vi "Joystick Drive Control.vi"(10 "Arcade Drive?":bool, 11 "Cluster In":T11) -> ()   [LabVIEW 2018]
uses:
  <vilib>/Rock Robotics/WPI/MotorControl/WPI_MotorControlDeviceRef.ctl
  <vilib>/Rock Robotics/WPI/MotorControl/WPI_MotorControlType.ctl
  <vilib>/Rock Robotics/SystemInterfaces/DIO/FPGA_DIOPWMChannel.ctl
  <vilib>/Rock Robotics/WPI/PWM/WPI_PWMDeadband.ctl
  <vilib>/Rock Robotics/SystemInterfaces/DIO/FPGA_DIOChannel.ctl
  <vilib>/Rock Robotics/WPI/Joystick/WPI_JoystickDevRef.ctl
  <vilib>/Rock Robotics/WPI/Joystick/WPI_JoystickDeviceEnum.ctl
  <vilib>/Rock Robotics/WPI/DriverStation/WPI_DriverStationRobotMode2.ctl
  <vilib>/Rock Robotics/WPI/RobotDrive/WPI_RobotDriveDevRef.ctl
  Vision States.ctl
  <vilib>/Rock Robotics/WPI/ThirdParty/Phoenix-LabVIEW/Motor Controller/Controls/CTRE_Phoenix_MotorControl_ControlMode.ctl
  Robot Global Data.vi
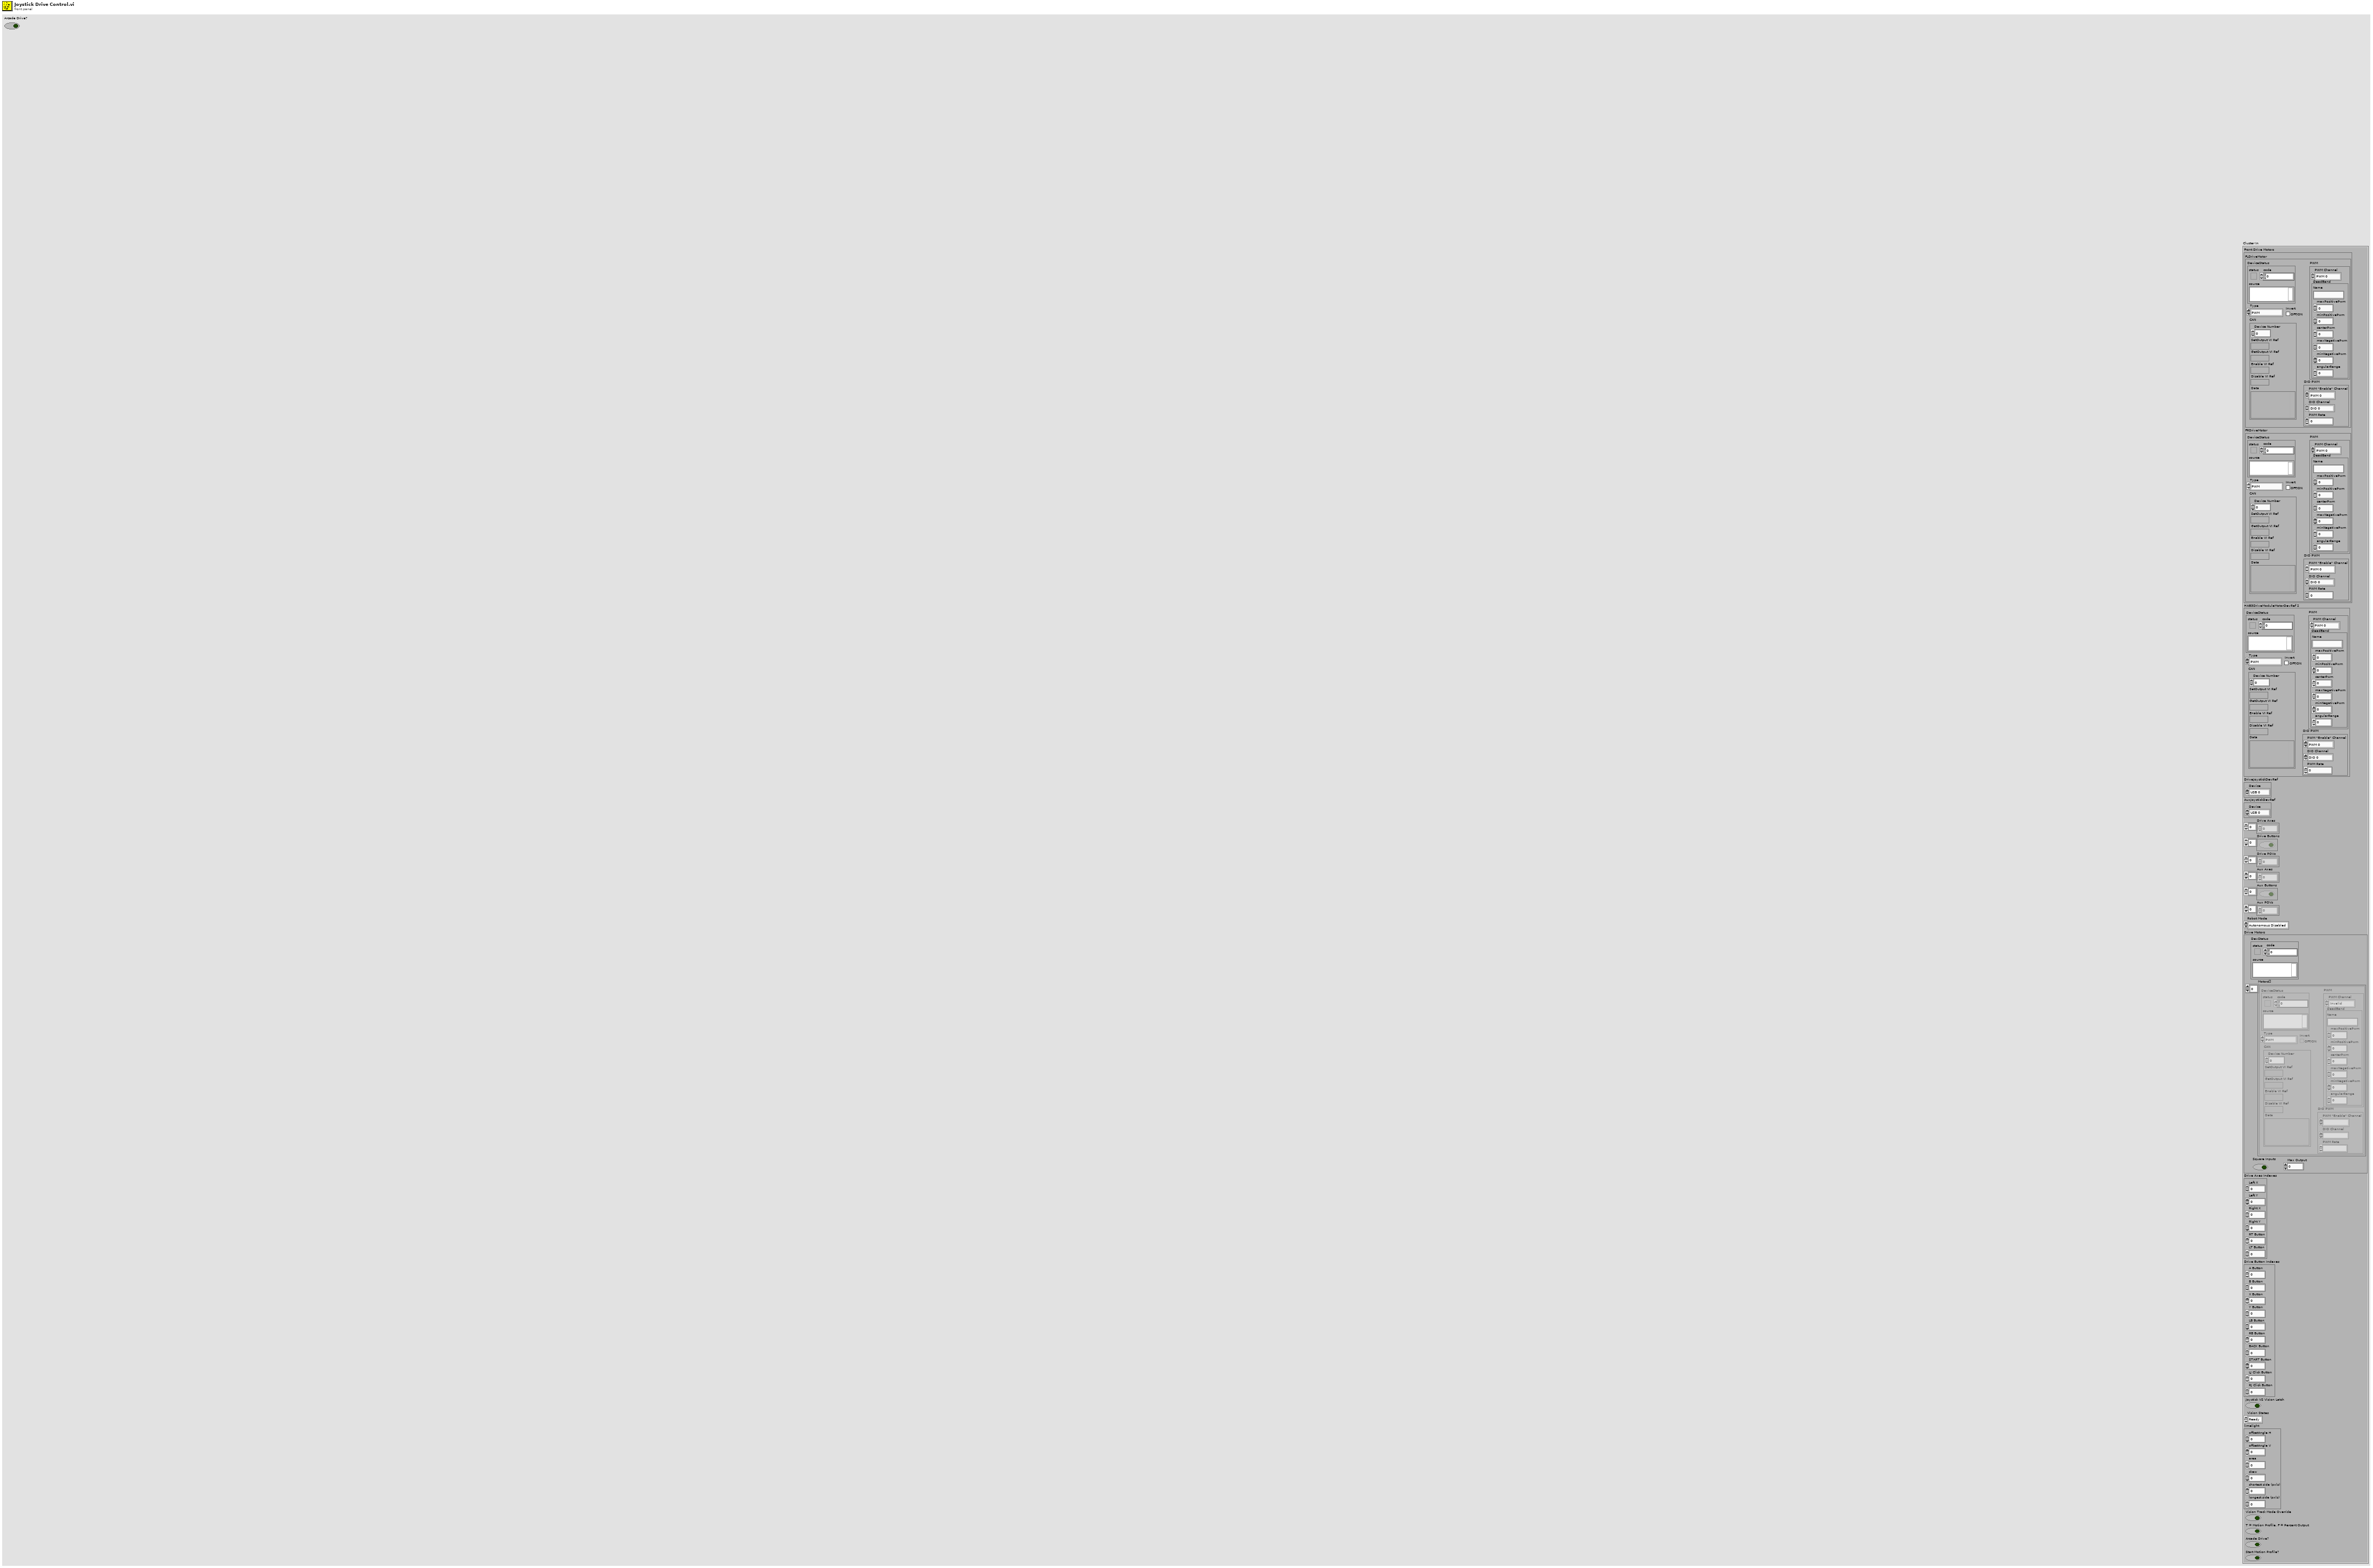
[diagram p1: front panel]
types:
  T1 = typedef "WPI_MotorControlDeviceRef.ctl" = cluster{"DeviceStatus":errorcluster, "Type":T2, "PWM":cluster{"PWM Channel":T3, "DeadBand":T4}, "CAN":cluster{"Device Number":u8, "SetOutput VI Ref":variant, "GetOutput VI Ref":variant, "Enable VI Ref":variant, "Disable VI Ref":variant, "Data":variant}, "Invert":bool, "DIO PWM":cluster{"PWM \"Enable\" Channel":T3, "DIOChannel":T5, "PWM Rate":dbl}}
  T2 = typedef "WPI_MotorControlType.ctl" = enum16{"PWM", "CAN", "DIO PWM"}
  T3 = typedef "FPGA_DIOPWMChannel.ctl" = enum8{"PWM 0", "PWM 1", "PWM 2", "PWM 3", "PWM 4", "PWM 5", "PWM 6", "PWM 7", "PWM 8", "PWM 9", "PWM MXP 0", "PWM MXP 1", "PWM MXP 2", "PWM MXP 3", "PWM MXP 4", "PWM MXP 5", "PWM MXP 6", "PWM MXP 7", "PWM MXP 8", "PWM MXP 9", "Invalid"}
  T4 = typedef "WPI_PWMDeadband.ctl" = cluster{"Name":string, "maxPositivePwm":i32, "minPositivePwm":i32, "centerPwm":i32, "maxNegativePwm":i32, "minNegativePwm":i32, "angularRange":u16}
  T5 = typedef "FPGA_DIOChannel.ctl" = enum8{"DIO 0", "DIO 1", "DIO 2", "DIO 3", "DIO 4", "DIO 5", "DIO 6", "DIO 7", "DIO 8", "DIO 9", "DIO MXP 0", "DIO MXP 1", "DIO MXP 2", "DIO MXP 3", "DIO MXP 4", "DIO MXP 5", "DIO MXP 6", "DIO MXP 7", "DIO MXP 8", "DIO MXP 9", "DIO MXP 10", "DIO MXP 11", "DIO MXP 12", "DIO MXP 13", "DIO MXP 14", "DIO MXP 15", "SPI Port CS1", "SPI Port CS2", "SPI Port CS3", "SPI Port MISO", "SPI Port MOSI", "Invalid"}
  T6 = typedef "WPI_JoystickDevRef.ctl" = cluster{"Device":T7}
  T7 = typedef "WPI_JoystickDeviceEnum.ctl" = enum16{"USB 0", "USB 1", "USB 2", "USB 3", "USB 4", "USB 5"}
  T8 = typedef "WPI_DriverStationRobotMode2.ctl" = enum16{"Autonomous Disabled", "Autonomous Enabled", "Teleop Disabled", "Teleop Enabled", "Disconnected", "Finish", "Test Disabled", "Test Enabled", "Emergency Stopped"}
  T9 = typedef "WPI_RobotDriveDevRef.ctl" = cluster{"DevStatus":errorcluster, "Motors[]":T1[], "Square Inputs":bool, "Max Output":dbl}
  T10 = typedef "Vision States.ctl" = enum16{"Ready", "Forward Until Target at Edge", "Vision Track"}
  T11 = cluster{"Front Drive Motors":cluster{"FLDriveMotor":T1, "FRDriveMotor":T1}, "HAB3DriveModuleMotorDevRef 2":T1, "DriveJoystickDevRef":T6, "AuxJoystickDevRef":T6, "Drive Axes":dbl[], "Drive Buttons":bool[], "Drive POVs":i16[], "Aux Axes":dbl[], "Aux Buttons":bool[], "Aux POVs":i16[], "Robot Mode":T8, "Drive Motors":T9, "Drive Axes Indexes":cluster{"Left X":i32, "Left Y":i32, "Right X":i32, "Right Y":i32, "RT Button":i32, "LT Button":i32}, "Drive Button Indexes":cluster{"A Button":i32, "B Button":i32, "X Button":i32, "Y Button":i32, "LB Button":i32, "RB Button":i32, "BACK Button":i32, "START Button":i32, "LJ Click Button":i32, "RJ Click Button":i32}, "Joystick VS Vision Latch":bool, "Vision States":T10, "limelight":cluster{"offsetAngle H":dbl, "offsetAngle V":dbl, "area":dbl, "skew":dbl, "shortest side (pxls)":dbl, "longest side (pxls)":dbl}, "Vision Track Mode Override":bool, "T = Motion Profile, F = Percent Output":bool, "Arcade Drive?":bool, "Start Motion Profile?":bool}
  T12 = typedef "CTRE_Phoenix_MotorControl_ControlMode.ctl" = u16
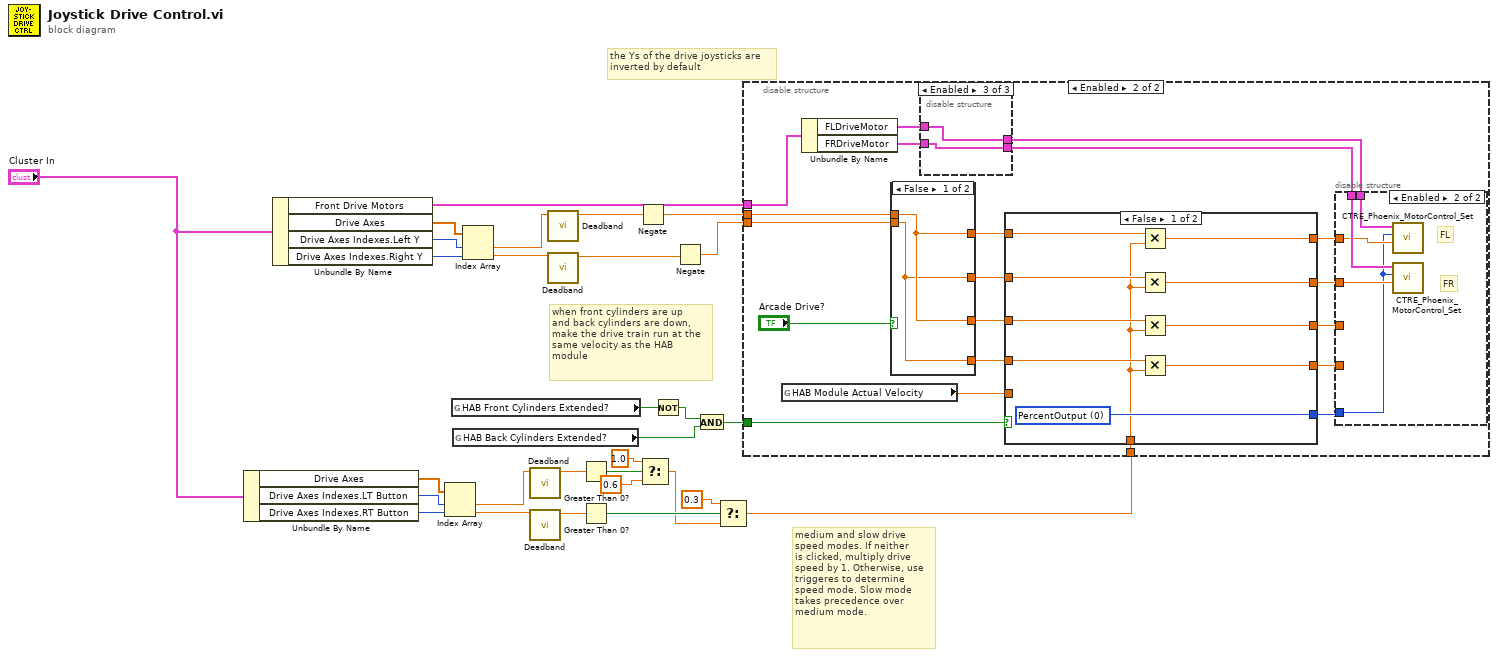
[diagram p0: block diagram]
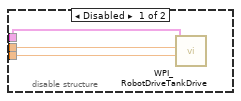
[diagram p2: hidden frame]
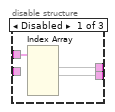
[diagram p3: hidden frame]
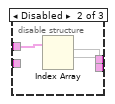
[diagram p4: hidden frame]
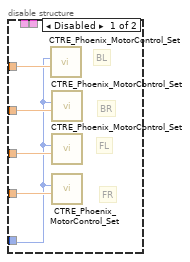
[diagram p5: hidden frame]
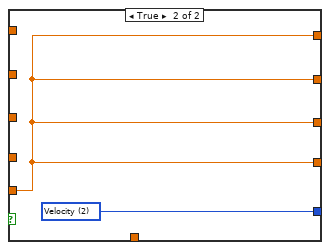
[diagram p7: hidden frame]
diagram:
  # "medium and slow drive\nspeed modes. If neither\nis clicked, multiply drive\nspeed by 1. Otherwise, use\ntriggeres to determine \nspeed mode. Slow mode\ntakes precedence over \nmedium mode."
  # "when front cylinders are up\nand back cylinders are down,\nmake the drive train run at the\nsame velocity as the HAB \nmodule"
  # "the Ys of the drive joysticks are \ninverted by default"
  n1 = Unbundle By Name("Cluster In") -> ("Drive Axes"=w13:dbl[], "Drive Axes Indexes.LT Button"=w14:i32, "Drive Axes Indexes.RT Button"=w15:i32)
  n2 = Unbundle By Name("Cluster In") -> ("Front Drive Motors"=w20:cluster{"FLDriveMotor":T1, "FRDriveMotor":T1}, "Drive Axes"=w21:dbl[], "Drive Axes Indexes.Left Y"=w22:i32, "Drive Axes Indexes.Right Y"=w23:i32)
  n3 = Index Array(array=w13, index #1=w14, index #2=w15) -> (element #1=w12:dbl, element #2=w16:dbl)
  n4 = global read "Robot Global Data.vi" "HAB Front Cylinders Extended?"() -> (w19:bool)
  n5 = global read "Robot Global Data.vi" "HAB Back Cylinders Extended?"() -> (w2:bool)
  n6 = Index Array(array=w21, index #1=w22, index #2=w23) -> (element #1=w26:dbl, element #2=w27:dbl)
  n7 = call "Deadband.vi"("Input"=w12) -> ("Output"=w11:dbl)  [unwired: 10 in]
  n8 = call "Deadband.vi"("Input"=w16) -> ("Output"=w10:dbl)  [unwired: 10 in]
  n9 = call "Deadband.vi"("Input"=w26) -> ("Output"=w29:dbl)  [unwired: 10 in]
  n10 = call "Deadband.vi"("Input"=w27) -> ("Output"=w28:dbl)  [unwired: 10 in]
  n11 = Greater Than 0?(x=w11) -> (x > 0?=w8:bool)
  n12 = Greater Than 0?(x=w10) -> (x > 0?=w9:bool)
  n13 = Negate(x=w29) -> (-x=w25:dbl)
  n14 = Select(t=1.0, s=w8, f=0.6) -> (s? t:f=w5:dbl)
  n15 = Not(x=w19) -> (.not. x?=w18:bool)
  n16 = Negate(x=w28) -> (-x=w24:dbl)
  n17 = And(x=w18, y=w2) -> (x .and. y?=w17:bool)
  n18 = Select(t=0.3, s=w9, f=w5) -> (s? t:f=w3:dbl)
  n19 = disable-structure shown="Enabled" {
    disable-tunnel: w25 -> [w32 w40]
    disable-tunnel: w24 -> [w31 w38]
    disable-tunnel: w20 -> [w30 w52]
    disable-tunnel: w17 -> [_ w46]
    disable-tunnel: w3 -> [_ w43]
    frame Disabled {
      n20 = call <vilib>:"WPI_RobotDriveTankDrive.vi"("Right axis value"=w31, "Left axis value"=w32, "RobotDriveDevRef"=w30) -> ()  [unwired: 6 in, 3 out]
    }
    frame Enabled {
      n21 = global read "Robot Global Data.vi" "HAB Module Actual Velocity"() -> (w45:dbl)
      n22 = Unbundle By Name(w52) -> ("FLDriveMotor"=w51:T1, "FRDriveMotor"=w33:T1)
      n23 = case shown="False" "Arcade Drive?" {
        tunnel: [w77 w78] -> w41
        tunnel: w40 -> [w77 w78]
        tunnel: [w76 w78] -> w39
        tunnel: w38 -> [w76 _]
        tunnel: [w77 w78] -> w37
        tunnel: [w76 w78] -> w36
        frame False {
        }
        frame True {
        }
      }
      n24 = disable-structure shown="Enabled" {
        disable-tunnel: w51 -> [w57 w60 w62]
        disable-tunnel: [w56 w59 w62] -> w35
        disable-tunnel: [w53 w58 w61] -> w34
        disable-tunnel: w33 -> [_ _ w61]
        frame Disabled {
          n25 = Index Array(array=w57) -> (element #1=w56, element #2=w53, element #3=w55, element #4=w54)  [unwired: 4 in]
        }
        frame Disabled {
          n26 = Index Array(array=w60) -> (element #1=w59, element #2=w58)  [unwired: 2 in]
        }
        frame Enabled {
        }
      }
      n27 = case shown="False" w46 {
        tunnel: w41 -> [w88 _]
        tunnel: [w80 w90] -> w50
        tunnel: w36 -> [w85 _]
        tunnel: [w83 w90] -> w49
        tunnel: w37 -> [w86 _]
        tunnel: [w82 w90] -> w48
        tunnel: w39 -> [w87 _]
        tunnel: [w81 w90] -> w47
        tunnel: w45 -> [_ w90]
        tunnel: [w84 w89] -> w44
        tunnel: w43 -> [w79 _]
        frame False {
          w84 = T12 0 items=["PercentOutput"=0, "Position"=1, "Velocity"=2, "Current"=3, "Follower"=5, "MotionProfile"=6, "MotionMagic"=7, "MotionProfileArc"=10, "Disabled"=15] ("Control Mode")
          n28 = Multiply(x=w88, y=w79) -> (x*y=w80:dbl)
          n29 = Multiply(x=w87, y=w79) -> (x*y=w81:dbl)
          n30 = Multiply(x=w86, y=w79) -> (x*y=w82:dbl)
          n31 = Multiply(x=w85, y=w79) -> (x*y=w83:dbl)
        }
        frame True {
          w89 = T12 2 items=["PercentOutput"=0, "Position"=1, "Velocity"=2, "Current"=3, "Follower"=5, "MotionProfile"=6, "MotionMagic"=7, "MotionProfileArc"=10, "Disabled"=15] ("Control Mode")
        }
      }
      n32 = disable-structure shown="Enabled" {
        disable-tunnel: w50 -> [w67 w73]
        disable-tunnel: w49 -> [w66 _]
        disable-tunnel: w48 -> [w65 _]
        disable-tunnel: w47 -> [w64 w72]
        disable-tunnel: w44 -> [w63 w71]
        disable-tunnel: w35 -> [_ w75]
        disable-tunnel: w34 -> [_ w74]
        frame Disabled {
          # "FR"
          # "FL"
          # "BR"
          # "BL"
          n33 = call <vilib>:"CTRE_Phoenix_MotorControl_Set.vi"("Output"=w67, "Control Mode"=w63) -> ()  [unwired: 8 in, 2 out]
          n34 = call <vilib>:"CTRE_Phoenix_MotorControl_Set.vi"("Output"=w64, "Control Mode"=w63) -> ("PhoenixMotorControlDevRef"=w68:T1)  [unwired: 7 in, 2 out]
          n35 = call <vilib>:"CTRE_Phoenix_MotorControl_Set.vi"("Output"=w65, "Control Mode"=w63) -> ("PhoenixMotorControlDevRef"=w70:T1)  [unwired: 7 in, 2 out]
          n36 = call <vilib>:"CTRE_Phoenix_MotorControl_Set.vi"("Output"=w66, "Control Mode"=w63) -> ("PhoenixMotorControlDevRef"=w69:T1)  [unwired: 7 in, 2 out]
        }
        frame Enabled {
          # "FR"
          # "FL"
          n37 = call <vilib>:"CTRE_Phoenix_MotorControl_Set.vi"("Output"=w73, "Control Mode"=w71, "PhoenixMotorControlDevRef"=w75) -> ()  [unwired: 7 in, 2 out]
          n38 = call <vilib>:"CTRE_Phoenix_MotorControl_Set.vi"("Output"=w72, "Control Mode"=w71, "PhoenixMotorControlDevRef"=w74) -> ()  [unwired: 7 in, 2 out]
        }
      }
    }
  }
